vi "target menu name.vi"(8 "error in":errorcluster, 11 "PLTarget cDAQ in":refnum<class "PLTarget cDAQ.lvclass">) -> (0 "error out":errorcluster, 2 "menu name":string, 3 "PLTarget cDAQ out":refnum<class "PLTarget cDAQ.lvclass">)   [LabVIEW 2013, in "PLTarget cDAQ.lvclass"]
uses:
  PLTarget cDAQ.lvclass
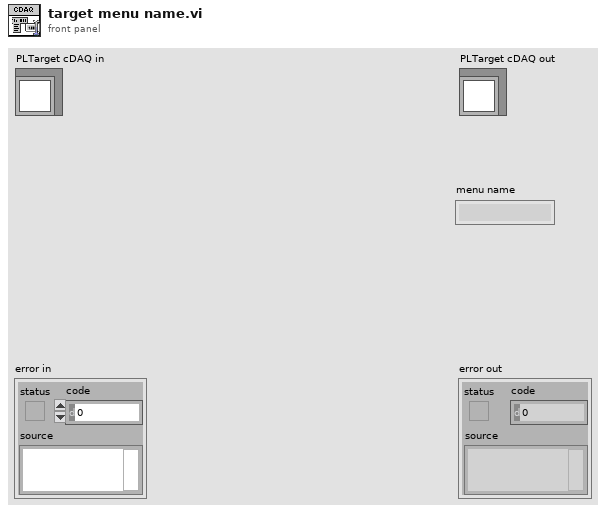
[diagram p1: front panel]
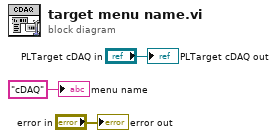
[diagram p0: block diagram]
diagram:
  "error out" <- "error in"
  "PLTarget cDAQ out" <- "PLTarget cDAQ in"
  "menu name" <- "cDAQ" ("menu name")
